vi "Constructor.vi"(11 "Worksheet":refnum<k7>) -> (3 "Excel Sheet out":refnum<class "Excel Sheet.lvclass">)   [LabVIEW 2016, in "Excel Sheet.lvclass"]
uses:
  Excel Sheet.lvclass
  Excel Sheet.lvclass/Excel Sheet.ctl
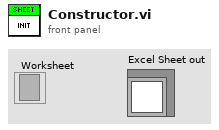
[diagram p1: front panel]
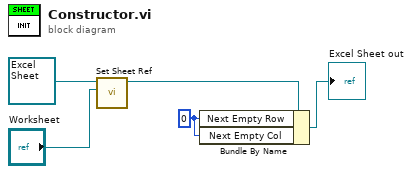
[diagram p0: block diagram]
diagram:
  w1 = 0 ("Next Empty Row")
  n1 = call-dynamic "Set Sheet Ref.vi"("Worksheet"="Worksheet", "Excel Sheet in"=refnum<class "Excel Sheet.lvclass"> refnum ("Excel Sheet.lvclass")) -> ("Excel Sheet out"=w3:refnum<class "Excel Sheet.lvclass">)  [unwired: 8 in, 1 out]
  n2 = Bundle By Name(cluster=w3, "Next Empty Row"=w1, "Next Empty Col"=w1) -> (→"Excel Sheet out":refnum<class "Excel Sheet.lvclass">)
